vi "FTW-Endpoint-BindToListener.vi"(0 "FTW-Endpoint In":refnum<class "FTW-Endpoint-TCP.lvclass">, 5 "Address":string, 11 "error in":errorcluster) -> (4 "FTW-Endpoint Out":refnum<class "FTW-Endpoint-TCP.lvclass">, 6 "Actual Address":string, 15 "error out":errorcluster)   [LabVIEW 2013, in "FTW-Endpoint-TCP.lvclass"]
uses:
  FTW-Endpoint-TCP.lvclass
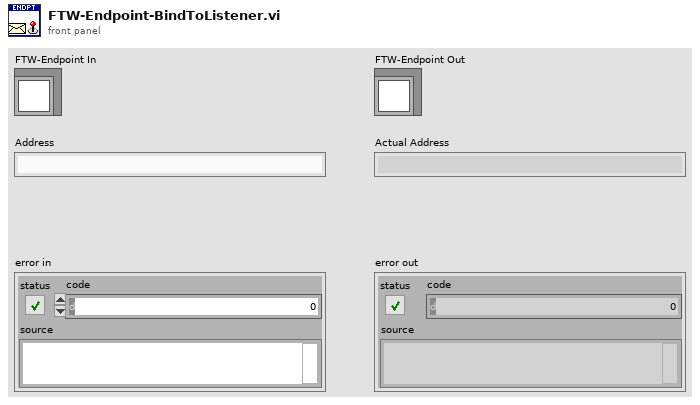
[diagram p1: front panel]
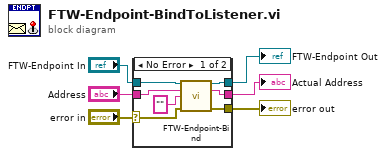
[diagram p0: block diagram]
diagram:
  n1 = case shown="No Error" "error in" {
    selector: "error in" -> [w12 w15]
    tunnel: [w11 w15] -> w6
    tunnel: [w10 w14] -> w5
    tunnel: "FTW-Endpoint In" -> [w13 w14]
    tunnel: "Address" -> [w7 _]
    tunnel: [w9 _] -> w1
    frame No Error {
      n2 = call-dynamic "FTW-Endpoint-Bind.vi"("FTW Endpoint"=w13, "Endpoint Address"=w7, "Requested Identity"="", "error in"=w12) -> ("FTW Endpoint out"=w10:refnum<class "FTW-Endpoint-TCP.lvclass">, "Actual Endpoint Address"=w9:string, "error out"=w11:errorcluster)  [unwired: 8 in, 1 out]
    }
    frame Error {
    }
  }
  "FTW-Endpoint Out" <- w5
  "error out" <- w6
  "Actual Address" <- w1
